vi "rsp_Get Settings.vi"(4 "Show in Debugger?":bool=TRUE, 6 "Message Priority":T1=enum."Normal", 8 "error in":errorcluster, 10 "Data in":T2, 11 "Settings Window in":refnum<class "Settings Window.lvclass">) -> (0 "error out":errorcluster, 3 "dup Settings Window out":refnum<class "Settings Window.lvclass">)   [LabVIEW 2023, in "Settings Window.lvclass"]
doc: "This VI sends a <b>Public API Response</b> message to a registered MHL case of the Caller of the Worker that owns this VI.\n---\nWorkers Public API Response"
uses:
  Settings Window.lvclass
  rsp_Get Settings.ctl
  Settings.ctl
  <vilib>/addons/_Workers/Library/Classes/Message/Priority.ctl
  Settings Window.lvclass/Settings Window.ctl
  <vilib>/Utility/error.llb/Error Cluster From Error Code.vi
  <vilib>/addons/_Workers/Library/Classes/Worker/Worker.lvclass
  <vilib>/addons/_Workers/Library/Classes/Message Queue/Message Queue.lvclass
  <vilib>/ErrorRing/Error Ring.xnode
  <vilib>/addons/_Workers/Library/Classes/Message/Message.lvclass
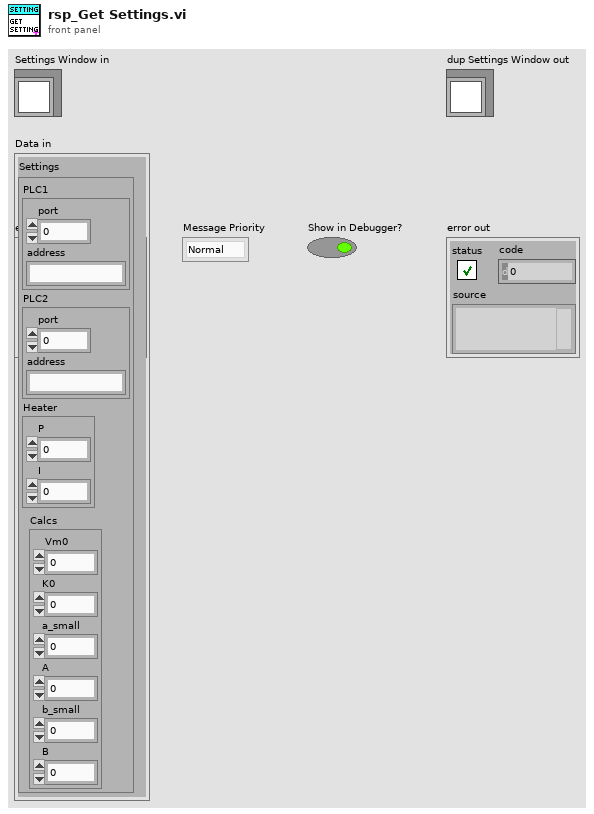
[diagram p1: front panel]
types:
  T1 = typedef "Workers.lvlib/Message.lvclass/Priority.ctl" = enum16{"Low", "Normal", "High"}
  T2 = typedef "Settings Window.lvclass/rsp_Get Settings.ctl" = cluster{"Settings":T3}
  T3 = typedef "Settings Window.lvclass/Settings.ctl" = cluster{"PLC1":cluster{"port":u16, "address":string}, "PLC2":cluster{"port":u16, "address":string}, "Heater":cluster{"P":dbl, "I":dbl}, "Calcs":cluster{"Vm0":dbl, "K0":dbl, "a_small":dbl, "A":dbl, "b_small":dbl, "B":dbl}}
  T4 = typedef "Workers.lvlib/Case Label.ctl" = string
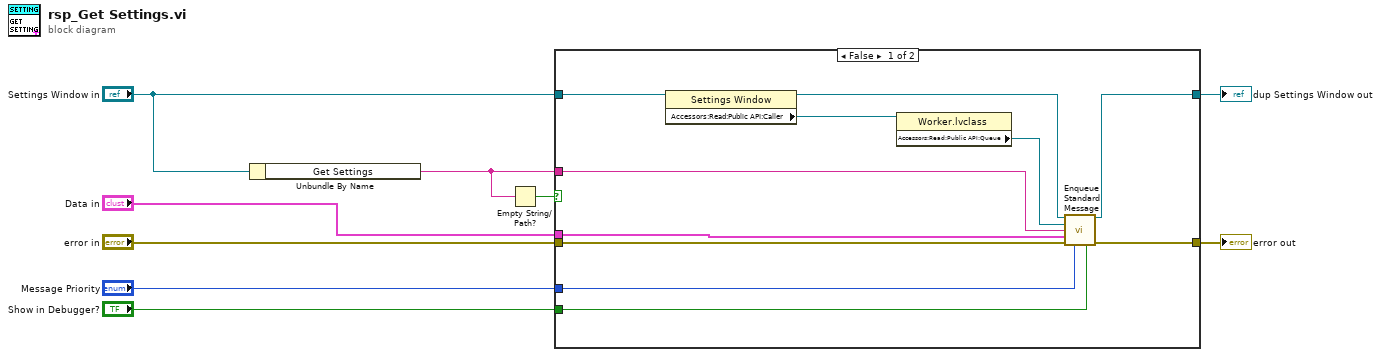
[diagram p0: block diagram]
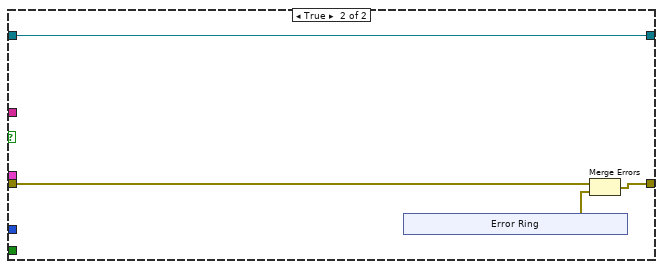
[diagram p2: hidden frame]
diagram:
  n1 = Unbundle By Name("Settings Window in") -> ("Get Settings"=w4:T4)
  n2 = Empty String/Path?(string/path=w4) -> (empty?=w5:bool)
  n3 = case shown="False" w5 {
    tunnel: "error in" -> [w20 w21]
    tunnel: [w19 w22] -> w8
    tunnel: "Data in" -> [w17 _]
    tunnel: [w18 w24] -> w6
    tunnel: "Settings Window in" -> [w14 w24]
    tunnel: w4 -> [w10 _]
    tunnel: "Show in Debugger?" -> [w16 _]
    tunnel: "Message Priority" -> [w15 _]
    frame False {
      n4 = property class="Settings Window"(reference=w14) -> (reference out=w13:refnum<class "Settings Window.lvclass">, "Accessors:Read:Public API:Caller"=w11:refnum<class "Worker.lvclass">)  [unwired: 1 in, 1 out]
      n5 = property class="Worker.lvclass"(reference=w11) -> ("Accessors:Read:Public API:Queue"=w12:refnum<class "Message Queue.lvclass">)  [unwired: 1 in, 2 out]
      n6 = call-dynamic "Enqueue Standard Message.vi"("Worker"=w13, "Message Queue"=w12, "Case Label"=w10, "Data"=w17, "error in (no error)"=w20, "Priority (Normal)"=w15, "Send Message to Debugger? (T)"=w16) -> ("dup Worker out"=w18:refnum<class "Settings Window.lvclass">, "error out"=w19:errorcluster)  [unwired: 7 in]
    }
    frame True {
      n7 = xnode "Error Ring"() -> ("error out"=w23:errorcluster)
      n8 = Merge Errors(w21, w23) -> (w22:errorcluster)
    }
  }
  "error out" <- w8
  "dup Settings Window out" <- w6
